vi "Selection.vi"(6 "Move Selection?":bool, 7 "Ants":refnum<class "Ants.lvclass">, 8 "error in (no error)":errorcluster, 9 "Ants Selection":T1, 10 "Current Coords":cluster{"x":i16, "y":i16}, 11 "Tools Paint in":refnum<class "Tools Paint.lvclass">) -> (0 "error out":errorcluster, 3 "Tools Paint out":refnum<class "Tools Paint.lvclass">)   [LabVIEW 2020, in "Tools Paint.lvclass"]
uses:
  Tools Paint.lvclass
  Ants/Ants.lvclass
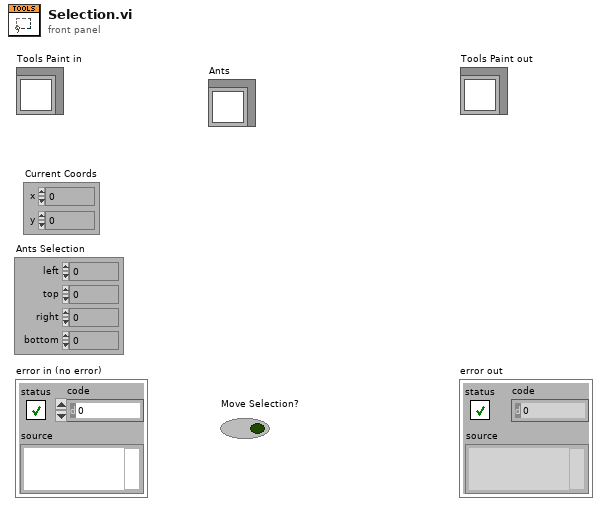
[diagram p1: front panel]
types:
  T1 = cluster{"left":i16, "top":i16, "right":i16, "bottom":i16}
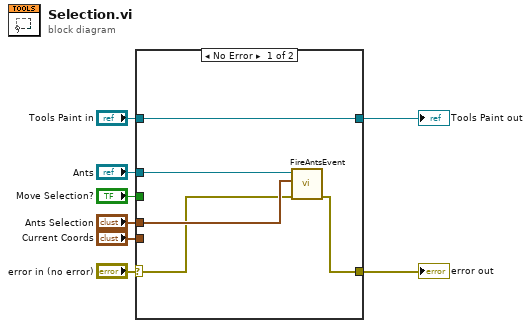
[diagram p0: block diagram]
diagram:
  n1 = case shown="No Error" "error in (no error)" {
    selector: "error in (no error)" -> [w10 w15]
    tunnel: [w11 w15] -> w7
    tunnel: [w13 w14] -> w5
    tunnel: "Tools Paint in" -> [w13 w14]
    tunnel: "Ants Selection" -> [w12 _]
    tunnel: "Current Coords" -> [_ _]
    tunnel: "Move Selection?" -> [_ _]
    tunnel: "Ants" -> [w9 _]
    frame No Error {
      n2 = call "FireAntsEvent.vi"("error in (no error)"=w10, "Rectangle (default: deselect)"=w12, "Ants in"=w9) -> ("error out"=w11:errorcluster)  [unwired: 1 in, 7 out]
    }
    frame Error {
    }
  }
  "error out" <- w7
  "Tools Paint out" <- w5
